vi "TxtFlash.vi"(6 "Index":i32=3, 7 "Adress":string, 8 "error in":errorcluster caption="错误输入", 9 "Model":string, 10 "ItemNames":string[][](array[string]), 11 "Path":string="Config\\data.ini") -> (0 "error out":errorcluster caption="错误输出")   [LabVIEW 2013]
panel:
  out "字符串":string
  out "添加的路径":path
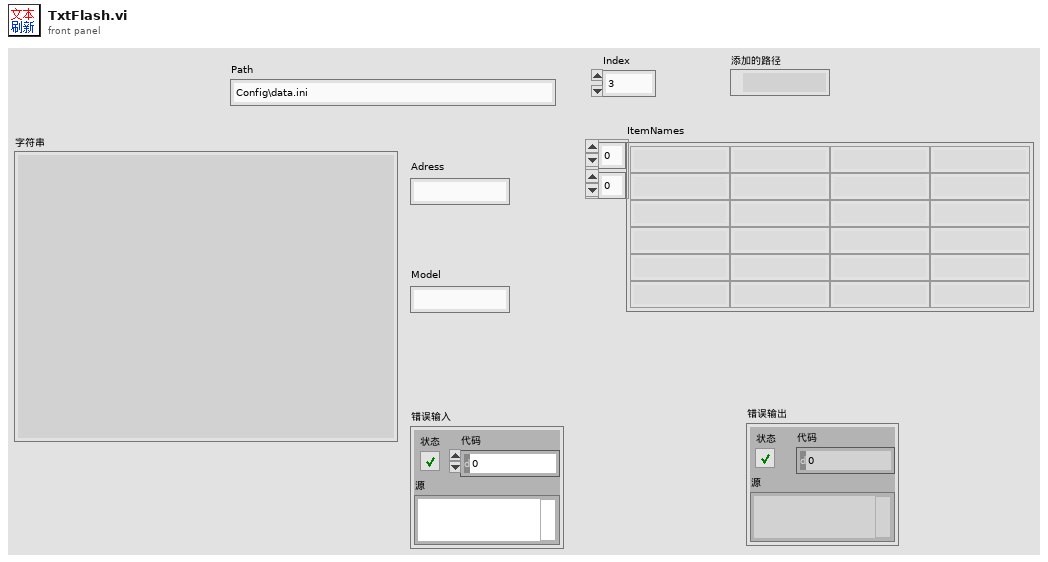
[diagram p1: front panel]
types:
  T1 = enum32{"invalid app kind", "Development System", "Run Time System", "Student Edition", "Embedded LabVIEW", "Evaluation", "Custom"}
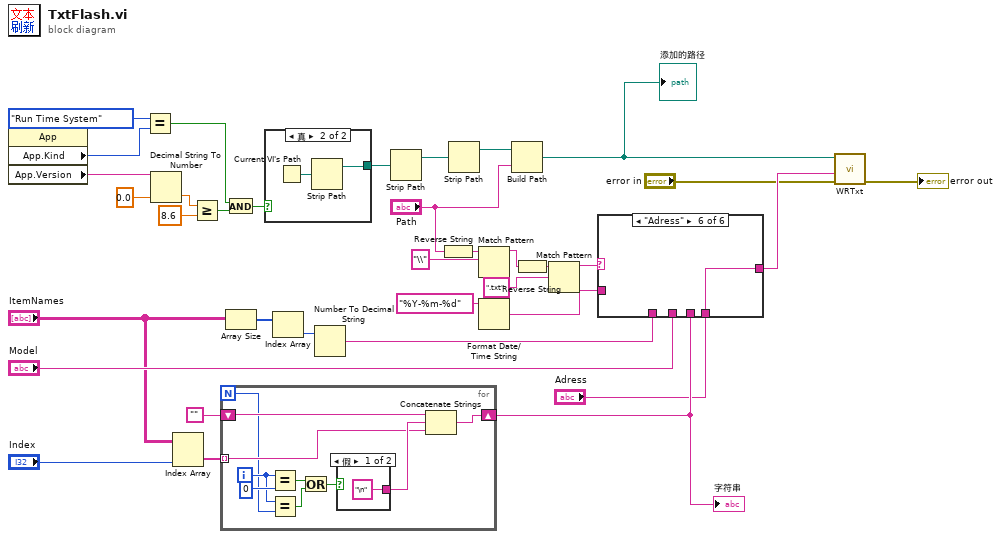
[diagram p0: block diagram]
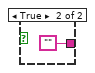
[diagram p2: hidden frame]
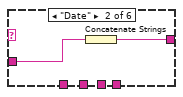
[diagram p4: hidden frame]
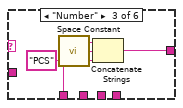
[diagram p5: hidden frame]
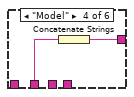
[diagram p6: hidden frame]
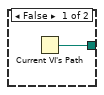
[diagram p8: hidden frame]
diagram:
  n1 = property class="App"() -> ("App.Kind"=w31:T1, "App.Version"=w32:string)  [unwired: 2 in, 2 out]
  n2 = Equal?(x=T1."Run Time System", y=w31) -> (x = y?=w28:bool)
  n3 = Decimal String To Number(string=w32, default (0L)=0.0 ("y")) -> (number=w34:dbl)  [unwired: 1 in, 1 out]
  n4 = Index Array(array="ItemNames", index (col)="Index") -> (element=w7:string[])  [unwired: 1 in]
  n5 = Greater Or Equal?(x=w34, y=8.6) -> (x >= y?=w27:bool)
  n6 = for {
    N -> [w36]
    tunnel: w7 -> [w38] mode=indexing
    shift-right: [w37] -> w2
    shift-left: "" -> [w45]
    i -> [w42]
    n7 = Equal?(x=w42, y=0) -> (x = y?=w44:bool)
    n8 = Equal?(x=w42, y=w36) -> (x = y?=w41:bool)
    n9 = Or(x=w44, y=w41) -> (x .or. y?=w40:bool)
    n10 = case shown="假" w40 {
      tunnel: ["\n" ""] -> w39
      frame False {
      }
      frame True {
      }
    }
    n11 = Concatenate Strings(w45, w39, w38) -> (w37:string)
  }
  "字符串" <- w2
  n12 = And(x=w28, y=w27) -> (x .and. y?=w29:bool)
  n13 = Array Size(array="ItemNames") -> (size(s)=w14:i32[])
  n14 = case shown="真" w29 {
    tunnel: [w48 w49] -> w25
    frame False {
      n15 = Current VI's Path() -> (path=w48:path)
    }
    frame True {
      n16 = Current VI's Path() -> (path=w50:path)
      n17 = Strip Path(path=w50) -> (stripped path=w49:path)  [unwired: 1 out]
    }
  }
  n18 = Index Array(array=w14) -> (element=w13:i32)  [unwired: 1 in]
  n19 = Number To Decimal String(number=w13) -> (decimal integer string=w12:string)  [unwired: 1 in]
  n20 = Strip Path(path=w25) -> (stripped path=w24:path)  [unwired: 1 out]
  n21 = Reverse String(1:"Path") -> (0:w5:string)
  n22 = Strip Path(path=w24) -> (stripped path=w26:path)  [unwired: 1 out]
  n23 = Match Pattern(string=w5, regular expression="\\") -> (before substring=w4:string)  [unwired: 1 in, 3 out]
  n24 = Format Date/Time String(time format string (%c)="%Y-%m-%d" ("时间格式字符串(%c)")) -> (date/time string=w17:string)  [unwired: 2 in]
  n25 = Build Path(base path=w26, name or relative path="Path") -> (appended path=w18:path)
  "添加的路径" <- w18
  n26 = Reverse String(1:w4) -> (0:w3:string)
  n27 = Match Pattern(string=w3, regular expression=".txt") -> (before substring=w19:string)  [unwired: 1 in, 3 out]
  n28 = case shown="\"Adress\"" w19 {
    tunnel: w17 -> [_ w52 _ _ _ _]
    tunnel: [_ w51 w56 w58 w59 w60] -> w16
    tunnel: w12 -> [_ _ w55 _ _ _]
    tunnel: "Model" -> [_ _ _ w57 _ _]
    tunnel: w2 -> [_ _ _ _ w59 _]
    tunnel: "Adress" -> [_ _ _ _ _ w60]
    frame "假", Default {
    }
    frame "Date" {
      n29 = Concatenate Strings(w52) -> (w51:string)
    }
    frame "Number" {
      n30 = call <vilib>:"Space Constant.vi"() -> ("String"=w54:string)
      n31 = Concatenate Strings(w55, w54, "PCS") -> (w56:string)
    }
    frame "Model" {
      n32 = Concatenate Strings(w57) -> (w58:string)
    }
    frame "SN" {
    }
    frame "Adress" {
    }
  }
  n33 = call "WRTxt.vi"("error in"="error in", "Text"=w16, "FilePath"=w18) -> ("error out"=→"error out":errorcluster)  [unwired: 8 in]
